vi "FPGA_PPG_resource_handler.vi"(0 "resource_in":refnum<visa-resource-name>, 2 "action":T2, 5 "error in (no error)":errorcluster) -> (14 "resource_out":refnum<visa-resource-name>, 16 "FPGA VI Reference Out":T1, 19 "error out":errorcluster)   [LabVIEW 2014, in "NI-FPGA_PPG_Driver.lvlib"]
doc: "Handles the FPGA resource. Please note, that you have to select a different bitfile, if you change to a FPGA target of different type. This has to be done in two places.\n- edit the properties of the \"FPGA_reference\" indicator on the front panel\n- edit the properties of the \"Open FPGA VI Reference\" VI in the \"SET\" case in the block diagram.\n\nContact: Falk Ziegler, eMail: info@lab-coding.de"
uses:
  NI-FPGA_PPG_Driver.lvlib
  FPGA_PPG_action_type.ctl
  FPGA_PPG_vi_ref.ctl
  <vilib>/FPGAPlugInAG/PXI-7852R/niLvFpga_Open_PXI-7852R.vi
  <vilib>/FPGAPlugInAG/PXI-7852R/niLvFpga_Close_PXI-7852R.vi
  <vilib>/rvi/interface/nirviOpenFPGA/nirviOpenFPGA.xnode
  FPGA Bitfiles/TiTaProj_COF_PPG_80MHz.lvbitx
  <vilib>/rvi/interface/nirviCloseFPGA/nirviCloseFPGA.xnode
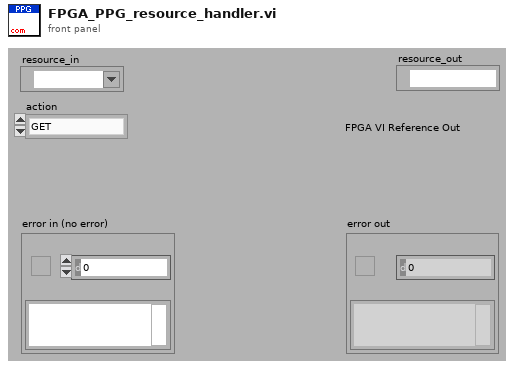
[diagram p1: front panel]
types:
  T1 = typedef "NI-FPGA_PPG_Driver.lvlib/FPGA_PPG_vi_ref.ctl" = refnum<k20>
  T2 = typedef "NI-FPGA_PPG_Driver.lvlib/FPGA_PPG_action_type.ctl" = enum16{"GET", "SET", "REMOVE"}
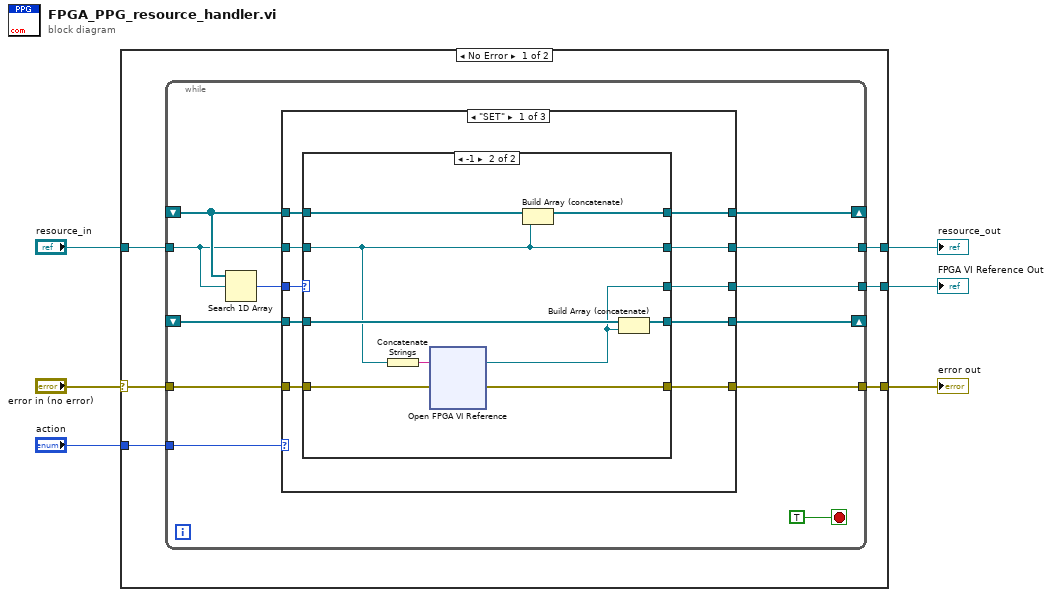
[diagram p0: block diagram]
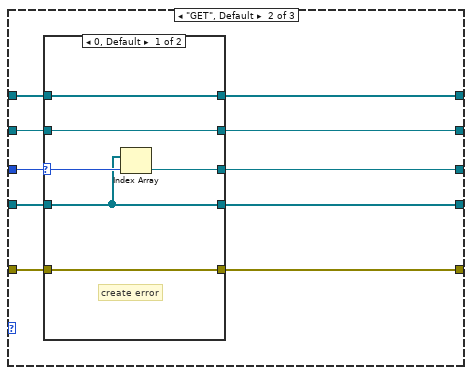
[diagram p3: hidden frame]
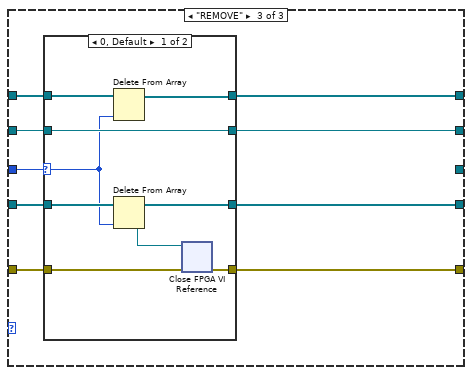
[diagram p5: hidden frame]
diagram:
  n1 = case shown="No Error" "error in (no error)" {
    selector: "error in (no error)" -> [w12 w90]
    tunnel: "action" -> [w11 _]
    tunnel: "resource_in" -> [w10 w91]
    tunnel: [w9 w91] -> w3
    tunnel: [w8 w90] -> w2
    tunnel: [w7 _] -> w1
    frame No Error {
      n2 = while {
        tunnel: w11 -> [w24]
        tunnel: w10 -> [w14]
        tunnel: w12 -> [w20]
        shift-right: [w22] -> _
        shift-left: _ -> [w17]
        tunnel: [w21] -> w9
        tunnel: [w19] -> w8
        shift-right: [w16] -> _
        shift-left: _ -> [w15]
        tunnel: [w13] -> w7
        stop <- TRUE stop-if-true
        n3 = Search 1D Array(1D array=w15, element=w14) -> (index of element=w23:i32)  [unwired: 1 in]
        n4 = case shown="\"SET\"" w24 {
          tunnel: w23 -> [w34 w57 w76]
          tunnel: w14 -> [w33 w56 w75]
          tunnel: w17 -> [w32 w55 w74]
          tunnel: [w28 w51 w70] -> w22
          tunnel: [w31 w54 w73] -> w21
          tunnel: w20 -> [w30 w53 w72]
          tunnel: [w29 w52 w71] -> w19
          tunnel: [w27 w50 w69] -> w16
          tunnel: w15 -> [w26 w49 w68]
          tunnel: [w25 w48 _] -> w13
          frame "SET" {
            n5 = case shown="-1" w34 {
              tunnel: w33 -> [w38 w41]
              tunnel: [w36 w47] -> w28
              tunnel: w32 -> [w36 w46]
              tunnel: [w38 w41] -> w31
              tunnel: w30 -> [w37 w43]
              tunnel: [w37 w42] -> w29
              tunnel: [w35 w45] -> w27
              tunnel: w26 -> [w35 w44]
              tunnel: [_ w40] -> w25
              frame 0, Default {
                # "create error"
              }
              frame -1 {
                n6 = Concatenate Strings ("Right-click and select Description and Tip")(w41) -> (w39:string)
                n7 = xnode "Open FPGA VI Reference"("error in"=w43, "resource name"=w39) -> ("FPGA VI Reference Out"=w40:T1, "error out"=w42:errorcluster)
                n8 = Build Array (concatenate)(w44, w41) -> (w45:refnum<visa-resource-name>[])
                n9 = Build Array (concatenate)(w46, w40) -> (w47:T1[])
              }
            }
          }
          frame "GET", Default {
            n10 = case shown="0, Default" w57 {
              selector: w57 -> [w60 _]
              tunnel: w56 -> [w63 w67]
              tunnel: [w59 w66] -> w51
              tunnel: w55 -> [w59 w66]
              tunnel: [w63 w67] -> w54
              tunnel: w53 -> [w62 w65]
              tunnel: [w62 w65] -> w52
              tunnel: [w61 w64] -> w50
              tunnel: w49 -> [w61 w64]
              tunnel: [w58 _] -> w48
              frame 0, Default {
                # "create error"
                n11 = Index Array(array=w59, index=w60) -> (element=w58:T1)
              }
              frame -1 {
                # "create error"
              }
            }
          }
          frame "REMOVE" {
            n12 = case shown="0, Default" w76 {
              selector: w76 -> [w77 _]
              tunnel: w75 -> [w85 w89]
              tunnel: [w83 w88] -> w70
              tunnel: w74 -> [w84 w88]
              tunnel: [w85 w89] -> w73
              tunnel: w72 -> [w82 w87]
              tunnel: [w81 w87] -> w71
              tunnel: [w78 w86] -> w69
              tunnel: w68 -> [w79 w86]
              frame 0, Default {
                n13 = Delete From Array(array=w79, index=w77) -> (array with subset deleted=w78:refnum<visa-resource-name>[])  [unwired: 1 in, 1 out]
                n14 = Delete From Array(array=w84, index=w77) -> (deleted portion=w80:T1, array with subset deleted=w83:T1[])  [unwired: 1 in]
                n15 = xnode "Close FPGA VI Reference"("FPGA VI Reference In"=w80, "error in"=w82) -> ("error out"=w81:errorcluster)
              }
              frame -1 {
                # "create error"
              }
            }
          }
        }
      }
    }
    frame Error {
    }
  }
  "error out" <- w2
  "resource_out" <- w3
  "FPGA VI Reference Out" <- w1
